vi "Terminal-DriverSystem-Getter.vi"(8 "error in (no error)":errorcluster caption="错误输入（无错误）", 11 "read operation timeout (ms)":i32=5000 caption="读操作超时（5000毫秒）") -> (0 "error out":errorcluster caption="错误输出", 3 "设备信息":T1)   [LabVIEW 2014]
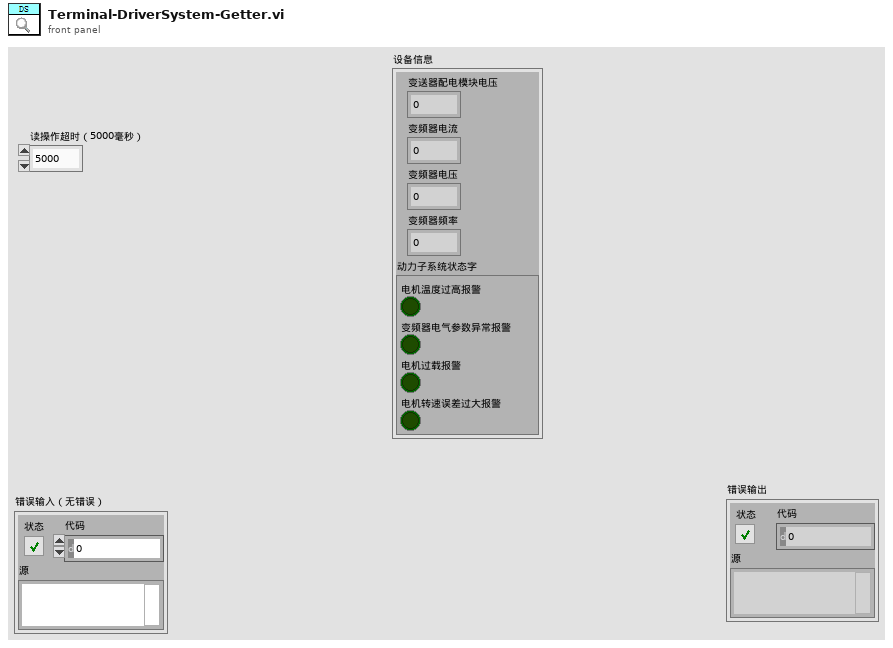
[diagram p1: front panel]
types:
  T1 = cluster{"变送器配电模块电压":u16, "变频器电流":u16, "变频器电压":u16, "变频器频率":u16, "动力子系统状态字":cluster{"电机温度过高报警":bool, "变频器电气参数异常报警":bool, "电机过载报警":bool, "电机转速误差过大报警":bool}}
  T2 = cluster{"电机温度过高报警":bool, "变频器电气参数异常报警":bool, "电机过载报警":bool, "电机转速误差过大报警":bool}
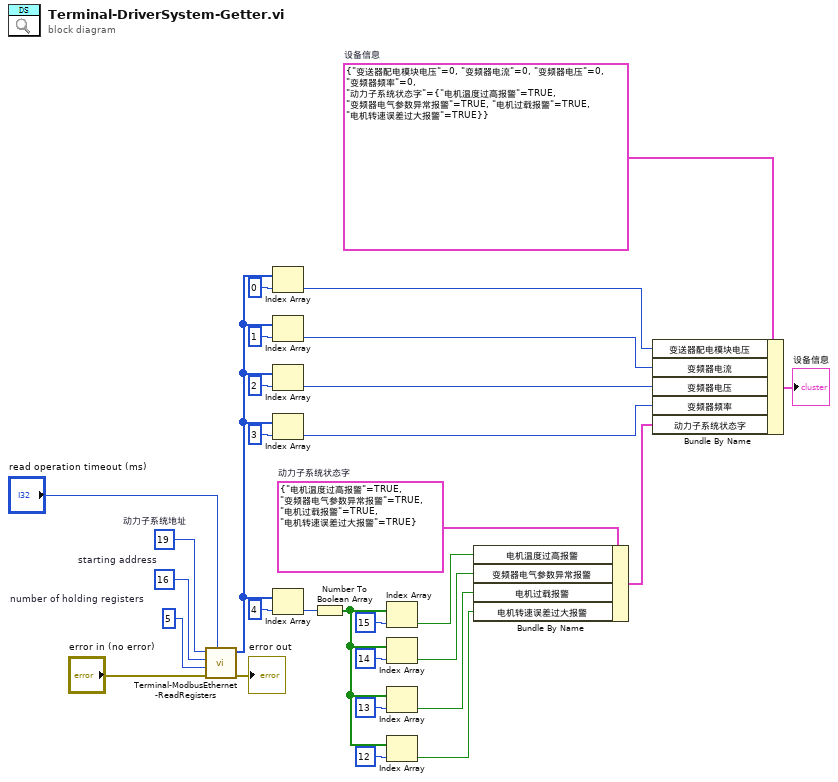
[diagram p0: block diagram]
diagram:
  w23 = T2 {"电机温度过高报警"=TRUE, "变频器电气参数异常报警"=TRUE, "电机过载报警"=TRUE, "电机转速误差过大报警"=TRUE}  # 动力子系统状态字
  w24 = T1 {"变送器配电模块电压"=0, "变频器电流"=0, "变频器电压"=0, "变频器频率"=0, "动力子系统状态字"={"电机温度过高报警"=TRUE, "变频器电气参数异常报警"=TRUE, "电机过载报警"=TRUE, "电机转速误差过大报警"=TRUE}}  # 设备信息
  w28 = u16 5  # number of holding registers
  w29 = u16 16  # starting address
  w30 = u8 19  # 动力子系统地址
  n1 = call "Terminal-ModbusEthernet-ReadRegisters.vi"("read operation timeout (ms)"="read operation timeout (ms)", "error in"="error in (no error)", "number of holding registers"=w28, "starting address"=w29, "unit ID"=w30) -> ("error out"=→"error out":errorcluster, "register values"=w12:u16[])  [unwired: 5 in]
  n2 = Index Array(array=w12, index=0 ("索引")) -> (element=w20:u16)
  n3 = Index Array(array=w12, index=1 ("索引")) -> (element=w15:u16)
  n4 = Index Array(array=w12, index=2 ("索引")) -> (element=w14:u16)
  n5 = Index Array(array=w12, index=3 ("索引")) -> (element=w13:u16)
  n6 = Index Array(array=w12, index=4 ("索引")) -> (element=w11:u16)
  n7 = Number To Boolean Array(number=w11) -> (Boolean array=w6:bool[])
  n8 = Index Array(array=w6, index=15 ("索引")) -> (element=w5:bool)
  n9 = Index Array(array=w6, index=14 ("索引")) -> (element=w4:bool)
  n10 = Index Array(array=w6, index=13 ("索引")) -> (element=w3:bool)
  n11 = Index Array(array=w6, index=12 ("索引")) -> (element=w2:bool)
  n12 = Bundle By Name(cluster=w23, "电机温度过高报警"=w5, "变频器电气参数异常报警"=w4, "电机过载报警"=w3, "电机转速误差过大报警"=w2) -> (w22:T2)
  n13 = Bundle By Name(cluster=w24, "变送器配电模块电压"=w20, "变频器电流"=w15, "变频器电压"=w14, "变频器频率"=w13, "动力子系统状态字"=w22) -> (→"设备信息":T1)
